vi "SMO.Example.GetPublicEventsRegistration.vi"(8 "error in (no error)":errorcluster, 11 "SMO.Example":refnum<class "SMO.TopLevel.lvclass">) -> (0 "error out":errorcluster, 2 "SMO.Example Public Events":refnum<event-registration>, 3 "SMO.Example out":refnum<class "SMO.TopLevel.lvclass">)   [LabVIEW 2013, in "SMO.TopLevel.lvclass"]
doc: "---------------------------------------------------------------\nJKI State Machine Objects™\nhttp://jki.net/state-machine-objects/\nCopyright (C) 2005-2015, JKI <info@jki.net>\nALL RIGHTS RESERVED"
uses:
  SMO.TopLevel.lvclass
  Typedefs/PublicEvents--Cluster.ctl
  Typedefs/DataChanged--EventData--Cluster.ctl
panel:
  # "For instructions on how to use the JKI State Machine Objects, examples and video tutorials, visit:\nhttp://jki.net/state-machine-objects/\n\nJKI State Machine Objects™\nhttp://jki.net/state-machine-objects/\nCopyright (C) 2005-2015, JKI <info@jki.net>\nALL RIGHTS RESERVED"
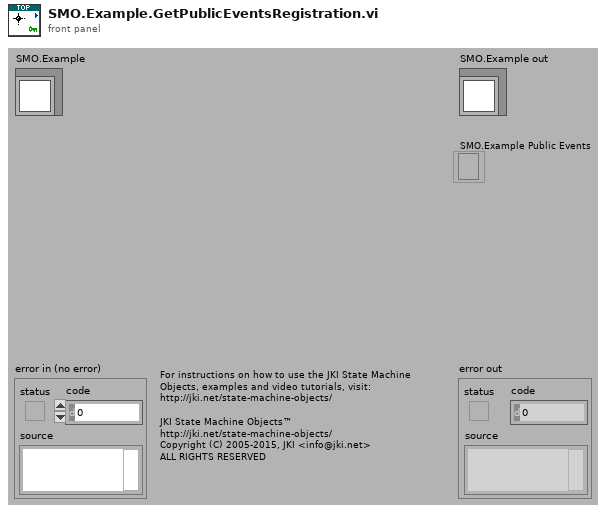
[diagram p1: front panel]
types:
  T1 = typedef "SMO.TopLevel.lvclass/PublicEvents--Cluster.ctl" = cluster{"Data Changed":refnum<user-event>}
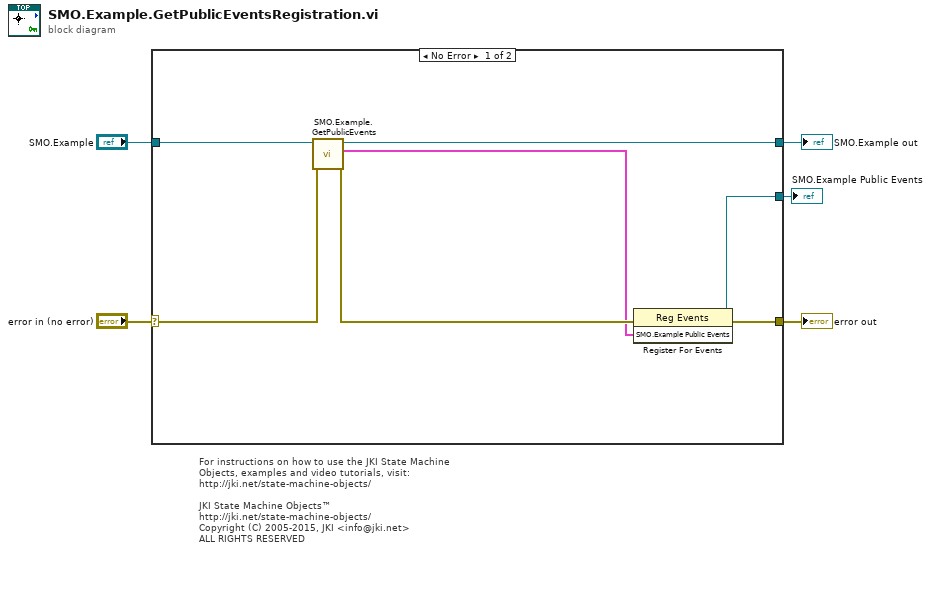
[diagram p0: block diagram]
diagram:
  # "For instructions on how to use the JKI State Machine Objects, examples and video tutorials, visit:\nhttp://jki.net/state-machine-objects/\n\nJKI State Machine Objects™\nhttp://jki.net/state-machine-objects/\nCopyright (C) 2005-2015, JKI <info@jki.net>\nALL RIGHTS RESERVED"
  n1 = case shown="No Error" "error in (no error)" {
    selector: "error in (no error)" -> [w9 w13]
    tunnel: "SMO.Example" -> [w10 w14]
    tunnel: [w12 w13] -> w4
    tunnel: [w6 w14] -> w3
    tunnel: [w11 _] -> w1
    frame No Error {
      n2 = call "SMO.Example.GetPublicEvents.vi"("error in (no error)"=w9, "SMO.Example"=w10) -> ("error out"=w8:errorcluster, "SMO.Example Public Events"=w7:T1, "SMO.Example out"=w6:refnum<class "SMO.TopLevel.lvclass">)  [unwired: 7 in]
      n3 = register-events(error in=w8, w7) -> (reference out=w11:refnum<event-registration>, error out=w12:errorcluster)  [unwired: 1 in]
    }
    frame Error {
    }
  }
  "error out" <- w4
  "SMO.Example out" <- w3
  "SMO.Example Public Events" <- w1
